vi "readTelemetryHardpointStatus.vi"(8 "error in (no error)":errorcluster, 10 "Parser":refnum<class "U8ArrayParserAutoIndexing.lvclass">, 11 "M1M3SAL in":refnum<class "M1M3SAL.lvclass">) -> (0 "error out":errorcluster, 2 "EventSummaryState":variant, 3 "M1M3SAL out":refnum<class "M1M3SAL.lvclass">)   [LabVIEW 2016, in "M1M3SupportCommunicator.lvlib" / "M1M3SAL.lvclass"]
uses:
  M1M3SAL.lvclass
  Common_RT_Utilities/U8ArrayParserAutoIndexing/U8ArrayParserAutoIndexing.lvclass
  DataTypes/Topics/TelemetryHardpointStatus.ctl
  DataTypes/Topics/Parts/Timestamp.ctl
  DataTypes/Topics/M1M3SupportTopics.lvlib
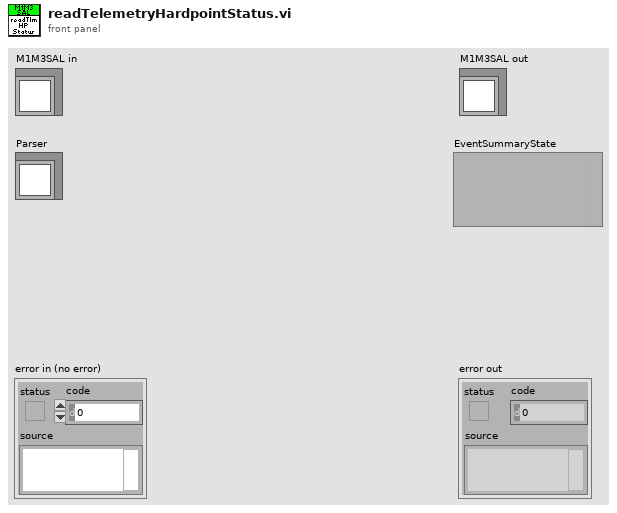
[diagram p1: front panel]
types:
  T1 = typedef "M1M3SupportTopics.lvlib/TelemetryHardpointStatus.ctl" = cluster{"Timestamp":T2, "Mode":u8[], "MajorFault":bool[], "MinorFault":bool[], "FaultOverridden":bool[], "WatchdogReset":bool[], "BrownoutDetected":bool[], "EventTrapReset":bool[], "MotorPowerFault":bool[], "SSRPowerFault":bool[], "AUXPowerFault":bool[], "SMCPowerFault":bool[]}
  T2 = typedef "M1M3SupportTopics.lvlib/Timestamp.ctl" = dbl
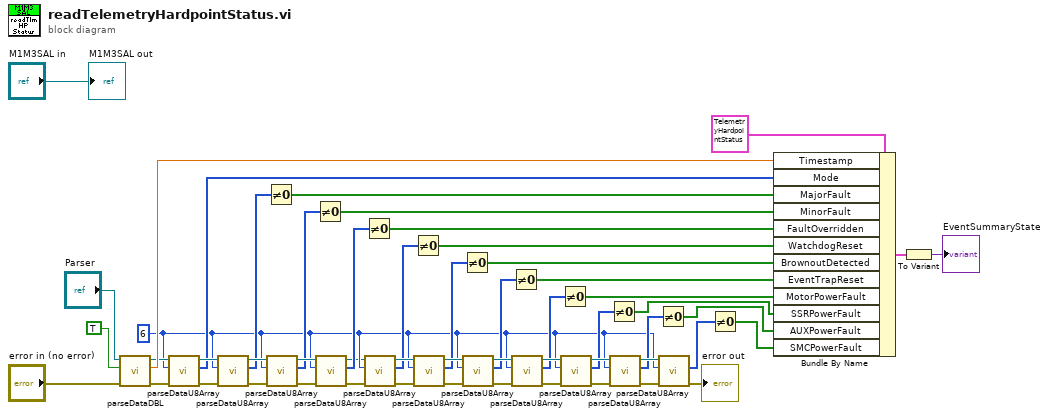
[diagram p0: block diagram]
diagram:
  w6 = 6 ("Length")
  n1 = call "parseDataDBL.vi"("error in (no error)"="error in (no error)", "OverrideSwapBytes"=TRUE, "U8ArrayParserAutoIndexing in"="Parser") -> ("error out"=w32:errorcluster, "Data"=w48:dbl, "U8ArrayParserAutoIndexing out"=w33:refnum<class "U8ArrayParserAutoIndexing.lvclass">)  [unwired: 6 in]
  n2 = call "parseDataU8Array.vi"("U8ArrayParserAutoIndexing in"=w33, "Length"=w6, "error in (no error)"=w32) -> ("U8ArrayParserAutoIndexing out"=w47:refnum<class "U8ArrayParserAutoIndexing.lvclass">, "Data"=w27:u8[], "error out"=w46:errorcluster)  [unwired: 5 in]
  n3 = call "parseDataU8Array.vi"("U8ArrayParserAutoIndexing in"=w47, "Length"=w6, "error in (no error)"=w46) -> ("U8ArrayParserAutoIndexing out"=w45:refnum<class "U8ArrayParserAutoIndexing.lvclass">, "Data"=w26:u8[], "error out"=w44:errorcluster)  [unwired: 5 in]
  n4 = Not Equal To 0?(x=w26) -> (x != 0?=w25:bool[])
  n5 = call "parseDataU8Array.vi"("U8ArrayParserAutoIndexing in"=w45, "Length"=w6, "error in (no error)"=w44) -> ("U8ArrayParserAutoIndexing out"=w31:refnum<class "U8ArrayParserAutoIndexing.lvclass">, "Data"=w24:u8[], "error out"=w30:errorcluster)  [unwired: 5 in]
  n6 = Not Equal To 0?(x=w24) -> (x != 0?=w23:bool[])
  n7 = call "parseDataU8Array.vi"("U8ArrayParserAutoIndexing in"=w31, "Length"=w6, "error in (no error)"=w30) -> ("U8ArrayParserAutoIndexing out"=w4:refnum<class "U8ArrayParserAutoIndexing.lvclass">, "Data"=w22:u8[], "error out"=w3:errorcluster)  [unwired: 5 in]
  n8 = Not Equal To 0?(x=w22) -> (x != 0?=w21:bool[])
  n9 = call "parseDataU8Array.vi"("U8ArrayParserAutoIndexing in"=w4, "Length"=w6, "error in (no error)"=w3) -> ("U8ArrayParserAutoIndexing out"=w43:refnum<class "U8ArrayParserAutoIndexing.lvclass">, "Data"=w20:u8[], "error out"=w42:errorcluster)  [unwired: 5 in]
  n10 = Not Equal To 0?(x=w20) -> (x != 0?=w19:bool[])
  n11 = call "parseDataU8Array.vi"("U8ArrayParserAutoIndexing in"=w43, "Length"=w6, "error in (no error)"=w42) -> ("U8ArrayParserAutoIndexing out"=w41:refnum<class "U8ArrayParserAutoIndexing.lvclass">, "Data"=w18:u8[], "error out"=w40:errorcluster)  [unwired: 5 in]
  n12 = Not Equal To 0?(x=w18) -> (x != 0?=w17:bool[])
  n13 = call "parseDataU8Array.vi"("U8ArrayParserAutoIndexing in"=w41, "Length"=w6, "error in (no error)"=w40) -> ("U8ArrayParserAutoIndexing out"=w39:refnum<class "U8ArrayParserAutoIndexing.lvclass">, "Data"=w16:u8[], "error out"=w38:errorcluster)  [unwired: 5 in]
  n14 = Not Equal To 0?(x=w16) -> (x != 0?=w15:bool[])
  n15 = call "parseDataU8Array.vi"("U8ArrayParserAutoIndexing in"=w39, "Length"=w6, "error in (no error)"=w38) -> ("U8ArrayParserAutoIndexing out"=w37:refnum<class "U8ArrayParserAutoIndexing.lvclass">, "Data"=w14:u8[], "error out"=w36:errorcluster)  [unwired: 5 in]
  n16 = Not Equal To 0?(x=w14) -> (x != 0?=w13:bool[])
  n17 = call "parseDataU8Array.vi"("U8ArrayParserAutoIndexing in"=w37, "Length"=w6, "error in (no error)"=w36) -> ("U8ArrayParserAutoIndexing out"=w29:refnum<class "U8ArrayParserAutoIndexing.lvclass">, "Data"=w12:u8[], "error out"=w28:errorcluster)  [unwired: 5 in]
  n18 = Not Equal To 0?(x=w12) -> (x != 0?=w11:bool[])
  n19 = call "parseDataU8Array.vi"("U8ArrayParserAutoIndexing in"=w29, "Length"=w6, "error in (no error)"=w28) -> ("U8ArrayParserAutoIndexing out"=w35:refnum<class "U8ArrayParserAutoIndexing.lvclass">, "Data"=w10:u8[], "error out"=w34:errorcluster)  [unwired: 5 in]
  n20 = Not Equal To 0?(x=w10) -> (x != 0?=w9:bool[])
  n21 = call "parseDataU8Array.vi"("U8ArrayParserAutoIndexing in"=w35, "Length"=w6, "error in (no error)"=w34) -> ("Data"=w8:u8[], "error out"=→"error out":errorcluster)  [unwired: 5 in, 1 out]
  n22 = Not Equal To 0?(x=w8) -> (x != 0?=w7:bool[])
  n23 = Bundle By Name(cluster=T1 {"Timestamp"=0.0, "Mode"=[], "MajorFault"=[], "MinorFault"=[], "FaultOverridden"=[], "WatchdogReset"=[], "BrownoutDetected"=[], "EventTrapReset"=[], "MotorPowerFault"=[], "SSRPowerFault"=[], "AUXPowerFault"=[], "SMCPowerFault"=[]} ("TelemetryHardpointStatus"), "Timestamp"=w48, "Mode"=w27, "MajorFault"=w25, "MinorFault"=w23, "FaultOverridden"=w21, "WatchdogReset"=w19, "BrownoutDetected"=w17, "EventTrapReset"=w15, "MotorPowerFault"=w13, "SSRPowerFault"=w11, "AUXPowerFault"=w9, "SMCPowerFault"=w7) -> (w52:T1)
  n24 = To Variant(anything=w52) -> (Variant=→"EventSummaryState":variant)
  "M1M3SAL out" <- "M1M3SAL in"
